vi "Destroy.vi"(8 "error in (no error)":errorcluster, 11 "Recipe Controller in":refnum<class "Recipe Controller.lvclass">) -> (0 "error out":errorcluster, 3 "Recipe Controller out":refnum<class "Recipe Controller.lvclass">)   [LabVIEW 2022 SP3, in "Recipe Controller.lvclass"]
uses:
  Recipe Controller.lvclass
  Recipe Controller.lvclass/Recipe Controller.ctl
  XY Stage/Process Actor/Process Framework/Interlock Q Class/Interlock Q Class.lvclass
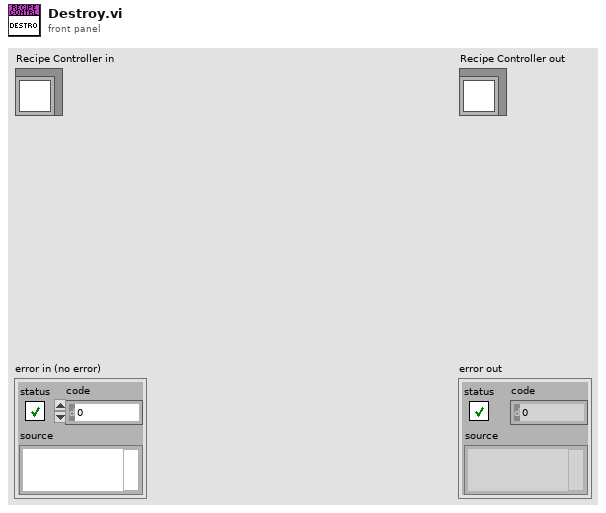
[diagram p1: front panel]
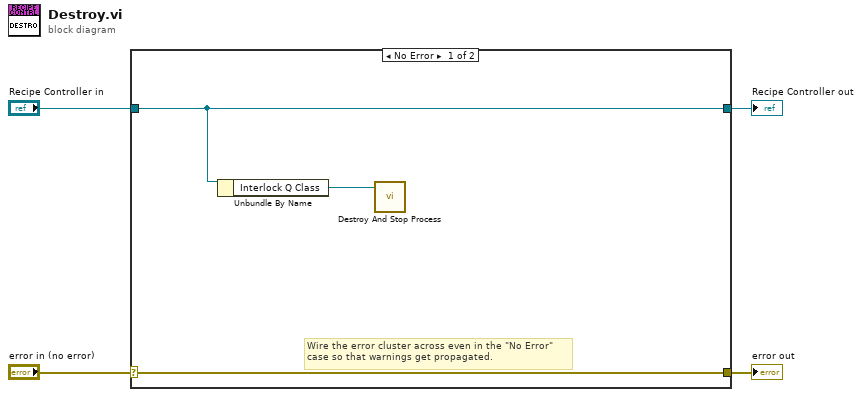
[diagram p0: block diagram]
diagram:
  n1 = case shown="No Error" "error in (no error)" {
    selector: "error in (no error)" -> [w7 w9]
    tunnel: [w7 w9] -> w3
    tunnel: [w6 w8] -> w1
    tunnel: "Recipe Controller in" -> [w6 w8]
    frame No Error {
      # "Wire the error cluster across even in the \"No Error\"\ncase so that warnings get propagated."
      n2 = Unbundle By Name(w6) -> ("Interlock Q Class"=w5:refnum<class "Interlock Q Class.lvclass">)
      n3 = call-dynamic "Destroy And Stop Process.vi"("Interlock Q Class in"=w5) -> ()  [unwired: 9 in, 2 out]
    }
    frame Error {
    }
  }
  "error out" <- w3
  "Recipe Controller out" <- w1
